vi "runLoopStop.vi"(8 "error in (no error)":errorcluster, 11 "Pixelfly in":refnum<class "PixelflySA.lvclass">) -> (0 "error out":errorcluster, 3 "Pixelfly out":refnum<class "PixelflySA.lvclass">)   [LabVIEW 2011, in "PixelflySA.lvclass"]
uses:
  PixelflySA.lvclass
  PixelflySA.lvclass/PixelflySA.ctl
  Tools/Filing/FileSystem/FileSystem.lvclass
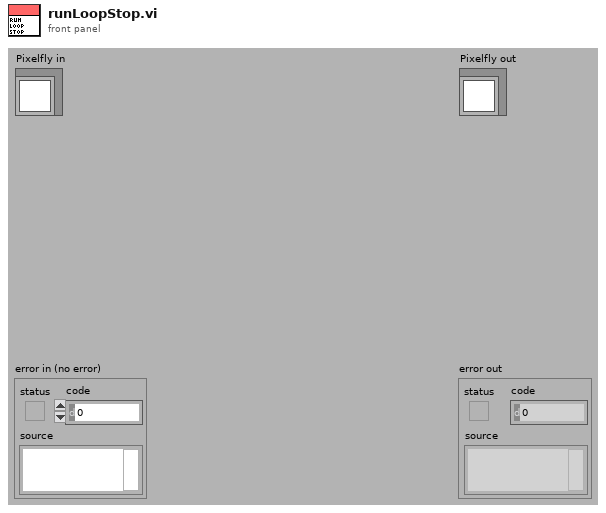
[diagram p1: front panel]
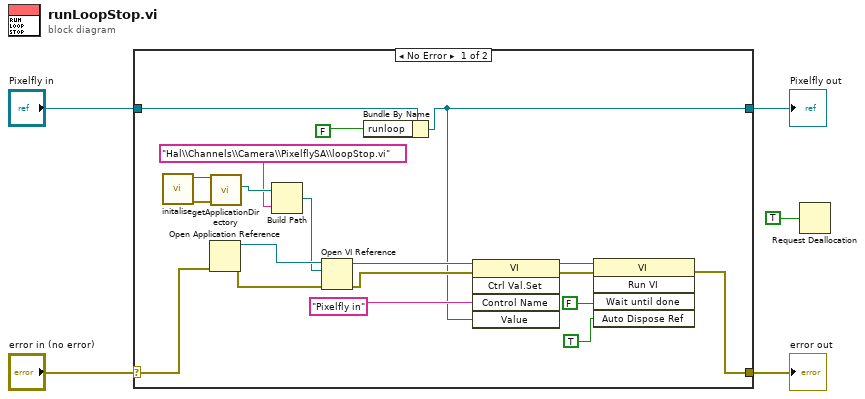
[diagram p0: block diagram]
diagram:
  n1 = case shown="No Error" "error in (no error)" {
    selector: "error in (no error)" -> [w17 w26]
    tunnel: [w9 w26] -> w4
    tunnel: [w7 w25] -> w2
    tunnel: "Pixelfly in" -> [w8 w25]
    frame No Error {
      n2 = call "initalise.vi"() -> ("error out"=w22:errorcluster, "FileSystem out"=w23:refnum<class "FileSystem.lvclass">)  [unwired: 10 in]
      n3 = Open Application Reference(8:w17) -> (0:w18:errorcluster, 3:w24:refnum<vi>)  [unwired: 3 in]
      n4 = call-dynamic "getApplicationDirectory.vi"("error in (no error)"=w22, "FileSystem.lvclass in"=w23) -> ("ApplicationDirectory"=w21:path)  [unwired: 7 in, 2 out]
      n5 = Build Path(base path=w21, name or relative path="Hal\\Channels\\Camera\\PixelflySA\\loopStop.vi") -> (appended path=w19:path)
      n6 = Open VI Reference(application reference (local)=w24, vi path=w19, error in (no error)=w18) -> (vi reference=w16:refnum<vi>, error out=w15:errorcluster)  [unwired: 3 in]
      n7 = Bundle By Name(cluster=w8, "runloop"=FALSE) -> (w7:refnum<class "PixelflySA.lvclass">)
      n8 = invoke class="VI" method="Ctrl Val.Set"(reference=w16, error in=w15, "Control Name"="Pixelfly in", "Value"=w7) -> (reference out=w12:refnum<vi>, error out=w13:errorcluster)  [unwired: 1 in, 3 out]
      n9 = invoke class="VI" method="Run VI"(reference=w12, error in=w13, "Wait until done"=FALSE, "Auto Dispose Ref"=TRUE) -> (error out=w9:errorcluster)  [unwired: 1 in, 4 out]
    }
    frame Error {
    }
  }
  "error out" <- w4
  "Pixelfly out" <- w2
  n10 = Request Deallocation(TRUE ("flag")) -> ()
